vi "OnResume.vi"(8 "error in (no error)":errorcluster, 11 "Game in":refnum<class "Game.lvclass">) -> (0 "error out":errorcluster, 3 "Game out":refnum<class "Game.lvclass">)   [LabVIEW 2019, in "RT_Game.lvlib" / "Game.lvclass"]
uses:
  Game.lvclass
  Game.lvclass/Game.ctl
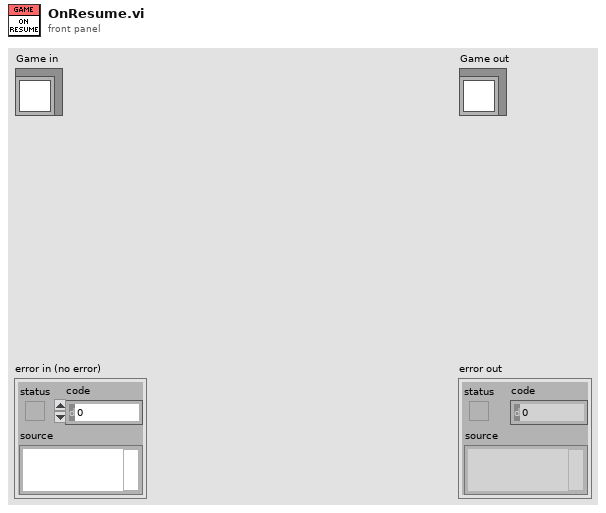
[diagram p1: front panel]
types:
  T1 = typedef "RT_Game.lvlib/Game.lvclass/States.ctl" = enum16{"Init", "Restart", "Menu", "Game", "Resume", "ToggleSingleplayer", "LoadNextGame", "ExitToMenu", "NewHighscore", "GameOver", "SlideOut"}
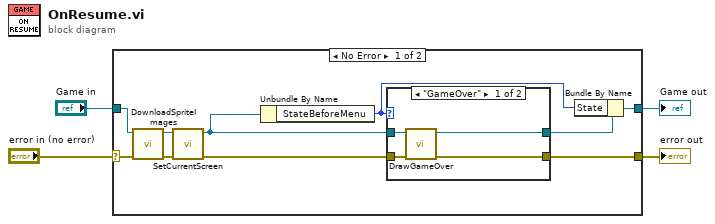
[diagram p0: block diagram]
diagram:
  n1 = case shown="No Error" "error in (no error)" {
    selector: "error in (no error)" -> [w14 w22]
    tunnel: [w10 w22] -> w3
    tunnel: [w12 w21] -> w1
    tunnel: "Game in" -> [w13 w21]
    frame No Error {
      n2 = call "DownloadSpriteImages.vi"("error in (no error)"=w14, "Game in"=w13) -> ("error out"=w11:errorcluster, "Game out"=w6:refnum<class "Game.lvclass">)  [unwired: 8 in]
      n3 = call-dynamic "SetCurrentScreen.vi"("error in (no error)"=w11, "Game in"=w6) -> ("error out"=w7:errorcluster, "Game out"=w5:refnum<class "Game.lvclass">)  [unwired: 8 in]
      n4 = Unbundle By Name(w5) -> ("StateBeforeMenu"=w8:T1)
      n5 = case shown="\"GameOver\"" w8 {
        tunnel: w7 -> [w18 w19]
        tunnel: [w17 w19] -> w10
        tunnel: [w16 w20] -> w9
        tunnel: w5 -> [w15 w20]
        frame "GameOver" {
          n6 = call "DrawGameOver.vi"("error in (no error)"=w18, "Game in"=w15) -> ("error out"=w17:errorcluster, "Game out"=w16:refnum<class "Game.lvclass">)  [unwired: 8 in]
        }
        frame Default {
        }
      }
      n7 = Bundle By Name(cluster=w9, "State"=w8) -> (w12:refnum<class "Game.lvclass">)
    }
    frame Error {
    }
  }
  "error out" <- w3
  "Game out" <- w1
